vi "get_IDs.vi"(8 "error in (no error)":errorcluster, 11 "PointLinkCollection in":refnum<class "PointLinkCollection.lvclass">) -> (0 "error out":errorcluster, 1 "IDs B":dbl[](array[numeric]), 2 "IDs A":dbl[](array[numeric]), 3 "PointLinkCollection out":refnum<class "PointLinkCollection.lvclass">, 4 "linked IDs":dbl[][](array[numeric]))   [LabVIEW 2010, in "PointLinkCollection.lvclass"]
uses:
  PointLinkCollection.lvclass
  PointLinkCollection.lvclass/PointLinkCollection.ctl
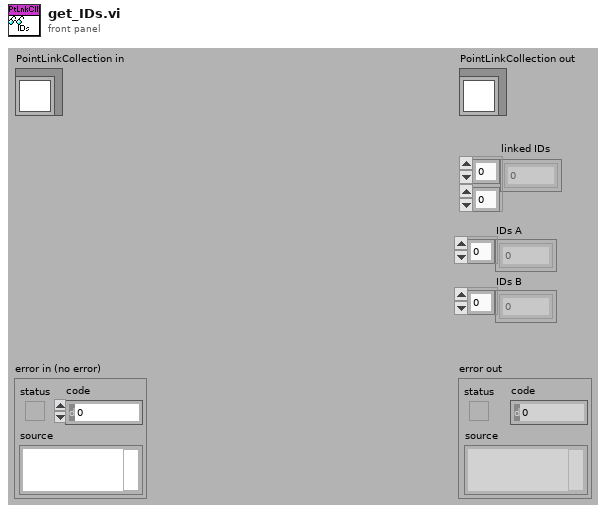
[diagram p1: front panel]
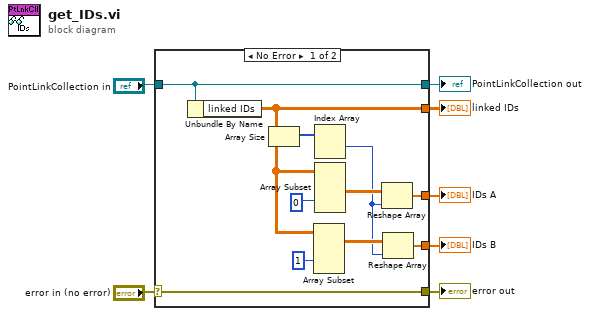
[diagram p0: block diagram]
diagram:
  n1 = case shown="No Error" "error in (no error)" {
    selector: "error in (no error)" -> [w18 w19]
    tunnel: [w18 w19] -> w6
    tunnel: [w17 w20] -> w4
    tunnel: "PointLinkCollection in" -> [w17 w20]
    tunnel: [w10 _] -> w3
    tunnel: [w9 _] -> w2
    tunnel: [w8 _] -> w1
    frame No Error {
      n2 = Unbundle By Name(w17) -> ("linked IDs"=w10:dbl[][])
      n3 = Array Size(array=w10) -> (size(s)=w14:i32[])
      n4 = Array Subset(array=w10, index (col)=1 ("index")) -> (w15:dbl[][])  [unwired: 3 in]
      n5 = Index Array(array=w14) -> (element #1=w13:i32)  [unwired: 2 in, 1 out]
      n6 = Array Subset(array=w10, index (col)=0 ("index")) -> (w16:dbl[][])  [unwired: 3 in]
      n7 = Reshape Array(w16, w13) -> (w9:dbl[])
      n8 = Reshape Array(w15, w13) -> (w8:dbl[])
    }
    frame Error {
    }
  }
  "error out" <- w6
  "PointLinkCollection out" <- w4
  "linked IDs" <- w3
  "IDs A" <- w2
  "IDs B" <- w1
